vi "close connection.vi"(8 "error in (no error)":errorcluster, 11 "SP in":refnum<class "Save messages PGserver.lvclass">) -> (0 "error out":errorcluster, 3 "SP out":refnum<class "Save messages PGserver.lvclass">)   [LabVIEW 2019, in "Save messages PGserver.lvclass"]
uses:
  Save messages PGserver.lvclass
  Save messages PGserver.lvclass/Save messages PGserver.ctl
  PostgreSQL2LabVIEW/libpqlv64/src/PQfinish.vi
  PostgreSQL2LabVIEW/libpqUtility64/libpqutility64.lvlib
  PostgreSQL2LabVIEW/libpqUtility/libpqutility.lvlib
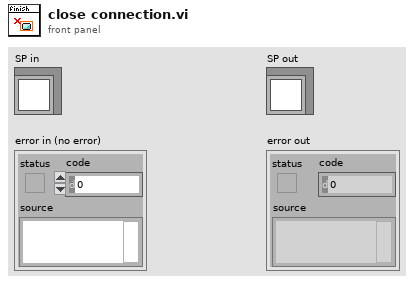
[diagram p1: front panel]
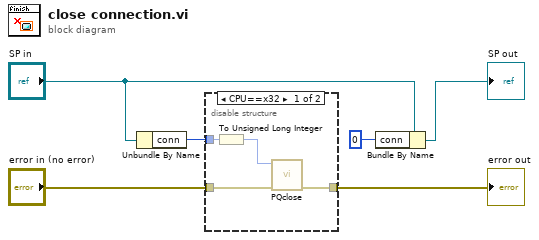
[diagram p0: block diagram]
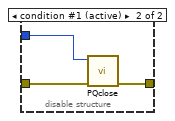
[diagram p2: hidden frame]
diagram:
  n1 = Unbundle By Name("SP in") -> ("conn"=w4:u64)
  n2 = disable-structure shown="CPU==x32" {
    disable-tunnel: w4 -> [w10 w13]
    disable-tunnel: "error in (no error)" -> [w9 w12]
    disable-tunnel: [w8 w11] -> w2
    frame condition #0 {
      n3 = To Unsigned Long Integer(number=w10) -> (unsigned 32bit integer=w7:u32)
      n4 = call "PQclose.vi"("error in (no error)"=w9, "conn"=w7) -> ("error out"=w8:errorcluster)  [unwired: 9 in]
    }
    frame condition #1 (active) {
      n5 = call "PQclose.vi"("error in (no error)"=w12, "conn"=w13) -> ("error out"=w11:errorcluster)  [unwired: 9 in]
    }
  }
  "error out" <- w2
  n6 = Bundle By Name(cluster="SP in", "conn"=u64 0) -> (→"SP out":refnum<class "Save messages PGserver.lvclass">)
